vi "Establish_Daqmx_v1.vi"(11 "DAQmx Device":tag="BoardTestStand") -> ()   [LabVIEW 2019]
panel:
  out "Loop Error?":errorcluster
  out "Instructional Message":string
  out "Unsuccesful Attempts to connect":i32
  in  "stop":bool
  out "error out":errorcluster
  in  "error in":errorcluster
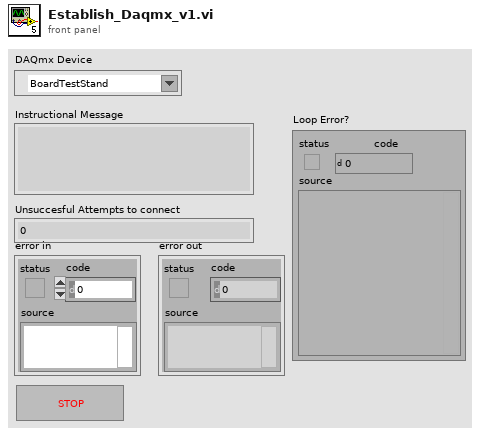
[diagram p1: front panel]
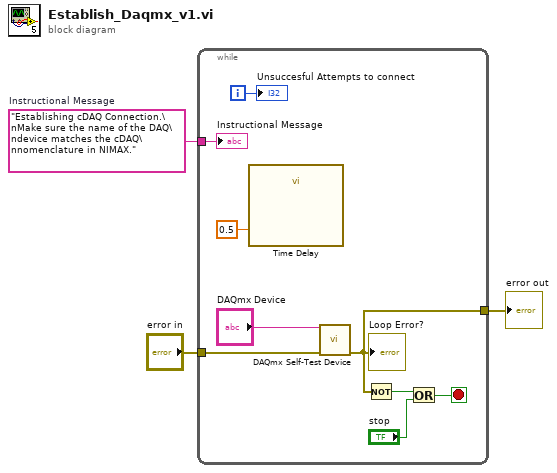
[diagram p0: block diagram]
diagram:
  w1 = "Establishing cDAQ Connection.\nMake sure the name of the DAQ\ndevice matches the cDAQ\nnomenclature in NIMAX."  # Instructional Message
  n1 = while {
    tunnel: "error in" -> [w12]
    tunnel: [w9] -> w2
    tunnel: w1 -> [w11]
    i -> [w10]
    stop <- w6 stop-if-true
    n2 = call "Time Delay"("Delay Time (s)"=0.5) -> ()  [unwired: 10 in, 1 out]
    n3 = call <vilib>:"DAQmx Self-Test Device.vi"("device in"="DAQmx Device", "error in"=w12) -> ("error out"=w9:errorcluster)  [unwired: 13 in]
    "Loop Error?" <- w9
    n4 = Not(x=w9) -> (.not. x?=w8:bool)
    n5 = Or(x=w8, y="stop") -> (x .or. y?=w6:bool)
    "Instructional Message" <- w11
    "Unsuccesful Attempts to connect" <- w10
  }
  "error out" <- w2
